vi "flashV6.vi"() -> ()   [LabVIEW 2017]
panel:
  in  "start":bool
  out "Current IP address":string
  in  "IP address list":string[](array[string])=["192.168.10.20", "192.168.10.22"]
  in  "回读":bool
  out "Current Progress":u32(slide)=3722240 scale=0.0..8559432.0
  out "error out":errorcluster={"status"=TRUE, "code"=4, "source"="Read from Binary File in flashV3.vi<APPEND>\nG:\\fpga_tdc\\FPGA\\TDC_2channel\\TOP.bin"}
  out "appended array":bool[](array[boolean])
  out "Process":u32=3722240
  in  "error in (no error)":errorcluster
  in  "Read (TRUE)":bool
  out "byte data":string
  out "Total size (in bytes)":i64=3722064
  in  "file path (use dialog)":path=path "G:/fpga_tdc/FPGA/SiTCP_410t/TDC_410t/TDC_410t.runs/impl_1/TOP.bin"
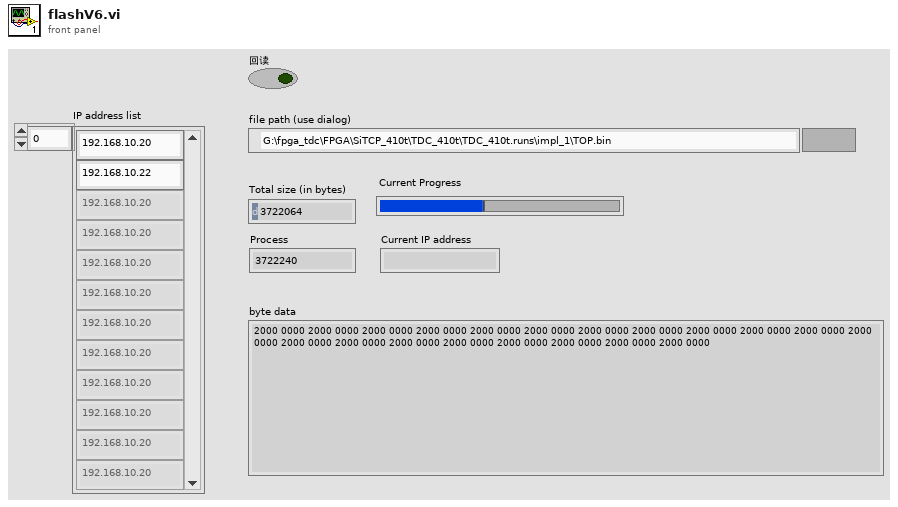
[diagram p1: front panel]
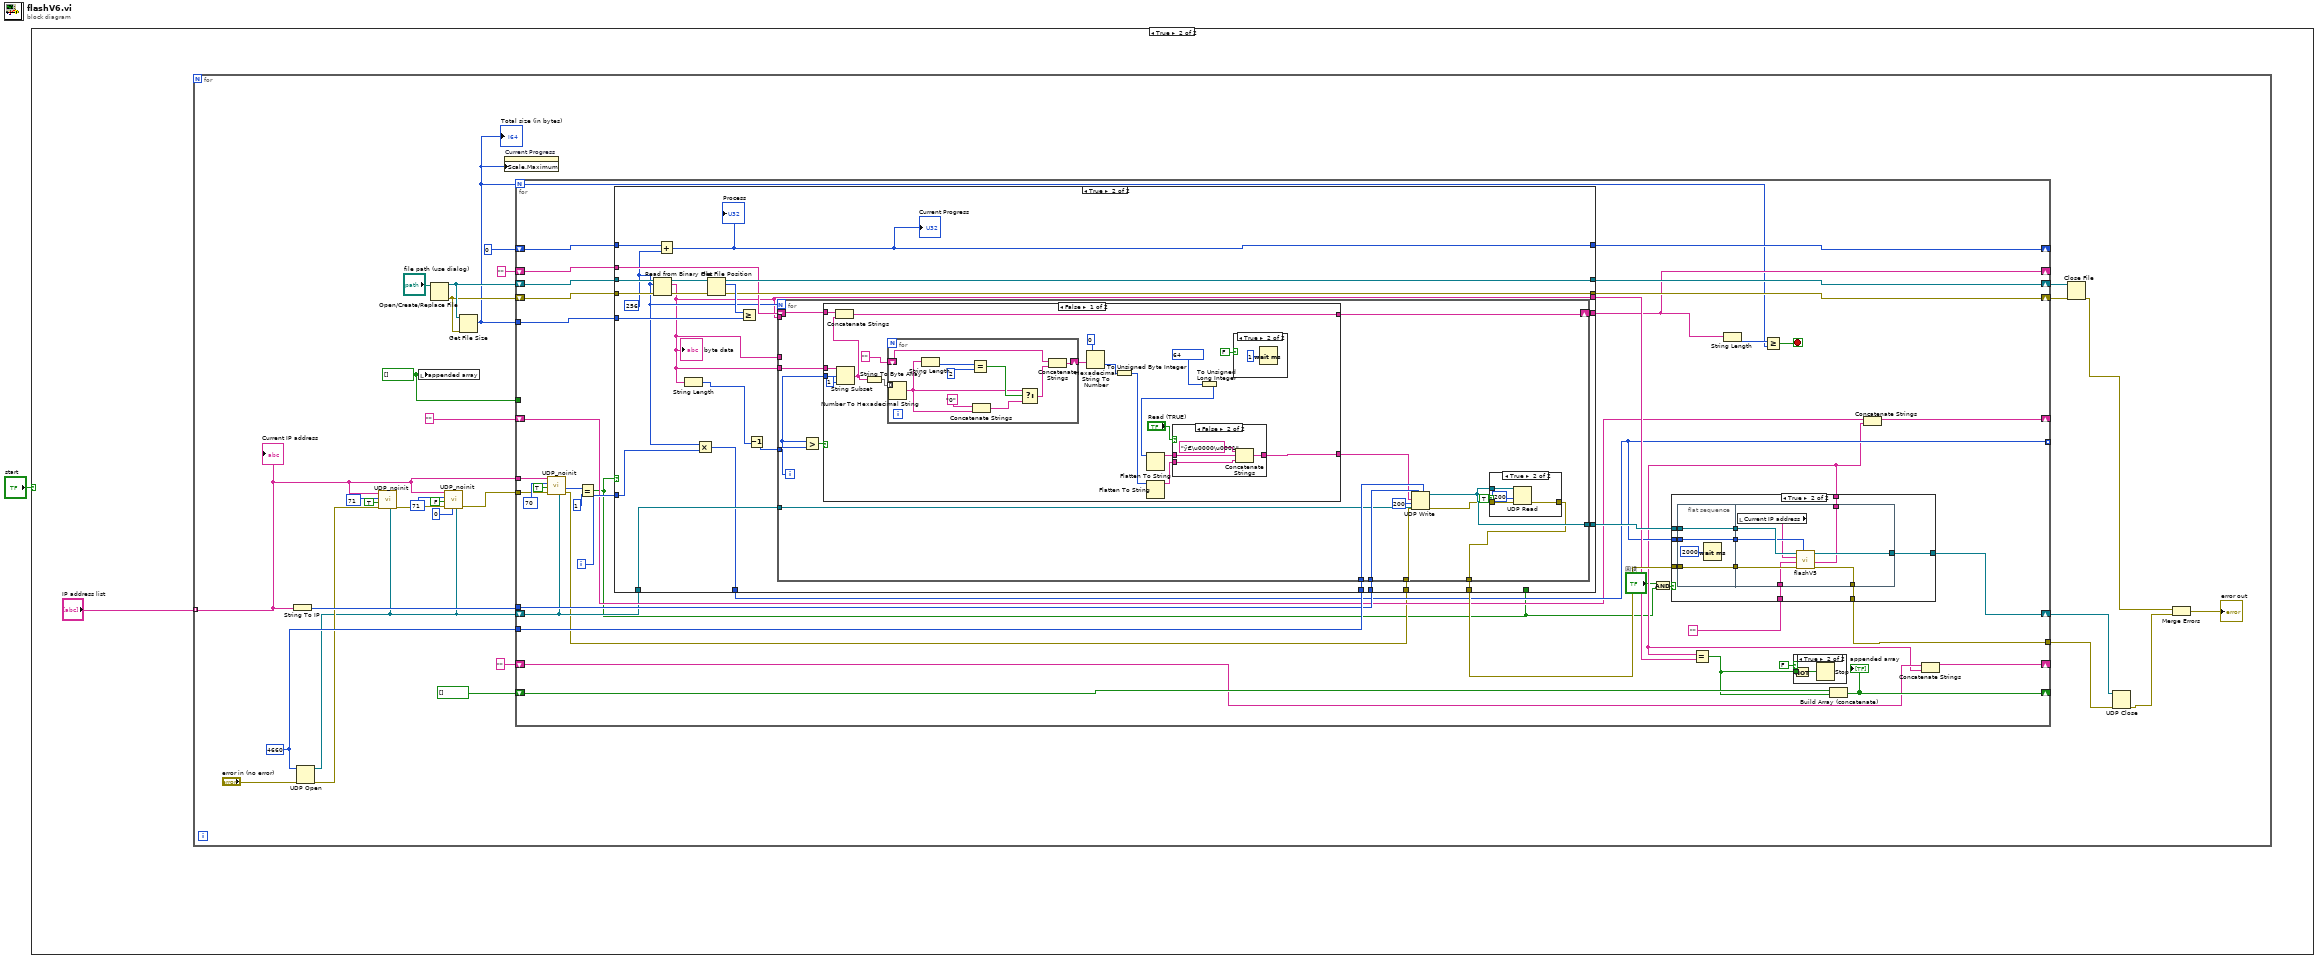
[diagram p0: block diagram]
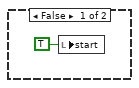
[diagram p2: hidden frame]
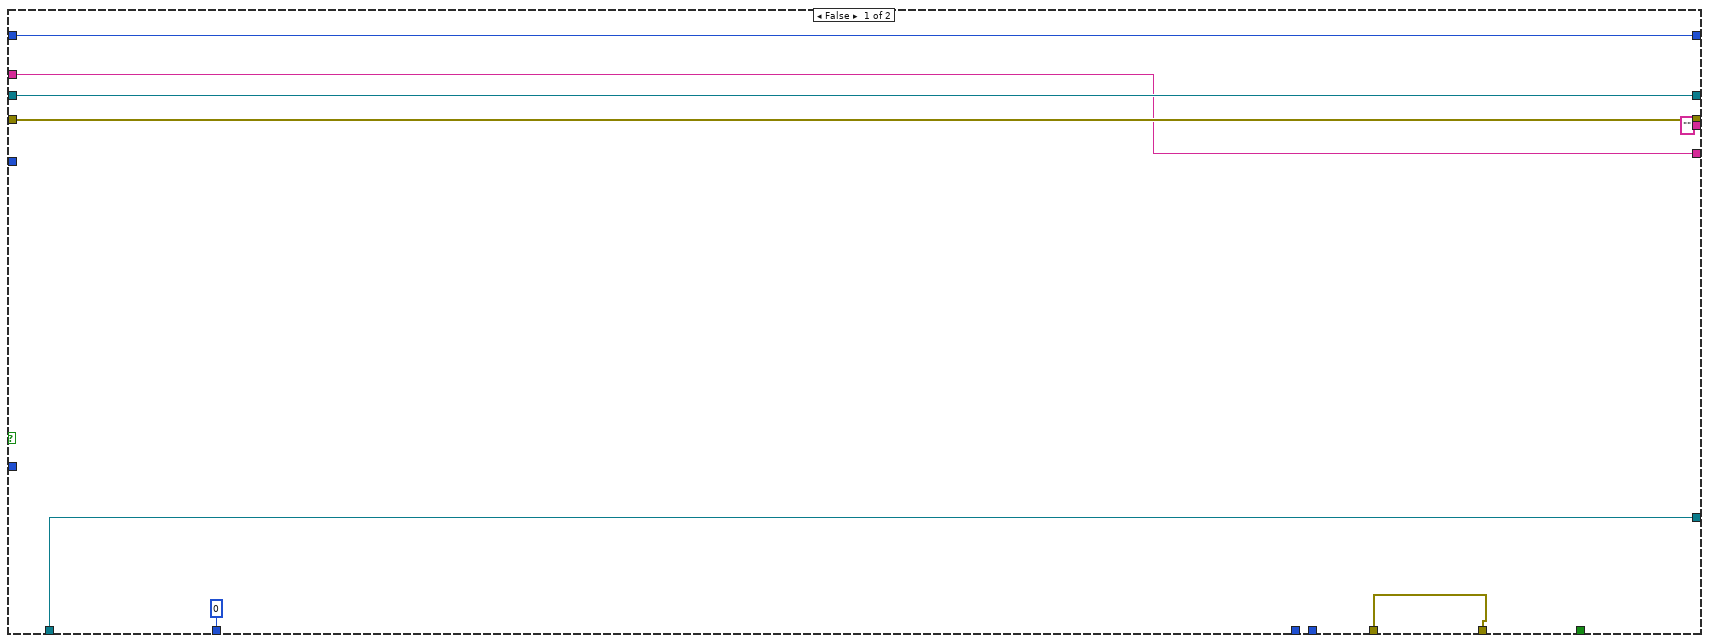
[diagram p3: hidden frame]
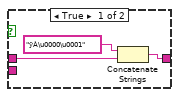
[diagram p5: hidden frame]
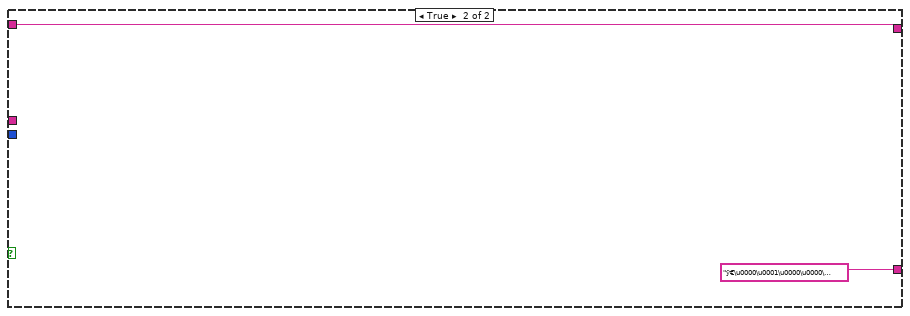
[diagram p7: hidden frame]
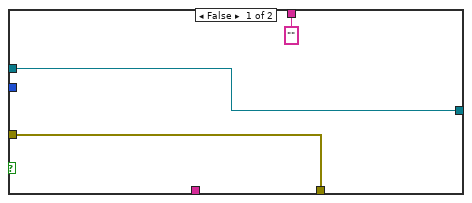
[diagram p8: hidden frame]
diagram:
  n1 = case shown="True" "start" {
    frame False {
      n2 = local write "start"(TRUE ("start")) -> ()
    }
    frame True {
      n3 = for {
        tunnel: "IP address list" -> [w13] mode=indexing
        w7 = bool[] [] ("appended array")
        w28 = u16 4660 ("UDP port")
        n4 = String To IP(1:w13) -> (0:w25:u32)
        n5 = UDP Open(8:"error in (no error)", 11:w28) -> (port=w10:refnum<k16>, 0:w15:errorcluster)  [unwired: 3 in, 1 out]
        n6 = call "UDP_noinit.vi"("connection ID"=w10, "error in (no error)"=w15, "Read (TRUE)"=TRUE, "Address"=u32 71, "IP address"=w13) -> ("error out"=w14:errorcluster)  [unwired: 3 in, 2 out]
        n7 = local write "appended array"(w7) -> ()
        n8 = Open/Create/Replace File(file path (use dialog)="file path (use dialog)") -> (refnum out=w32:refnum<file>, error out=w31:errorcluster)  [unwired: 5 in, 1 out]
        n9 = call "UDP_noinit.vi"("connection ID"=w10, "In"=u8 0, "error in (no error)"=w14, "Read (TRUE)"=FALSE, "Address"=u32 71, "IP address"=w13) -> ("error out"=w18:errorcluster)  [unwired: 2 in, 2 out]
        n10 = Get File Size(file=w32, error in=w31) -> (size (in bytes)=w8:i64)  [unwired: 2 out]
        "Total size (in bytes)" <- w8
        n11 = property on="Current Progress" class="Slide (strict)"("Scale.Maximum"=w8) -> ()  [unwired: 2 in, 2 out]
        n12 = for {
          N: w8 -> [w52]
          tunnel: w8 -> [w73]
          shift-right: [w72] -> w30
          shift-left: w31 -> [w74]
          shift-right: [w71] -> w29
          shift-left: w32 -> [w75]
          shift-right: [w54] -> _
          shift-left: "" -> [w70]
          tunnel: w28 -> [w67]
          tunnel: [w62] -> w26
          tunnel: w25 -> [w66]
          shift-right: [w64] -> w27
          shift-left: w10 -> [w41]
          shift-right: [w68] -> _
          shift-left: u32 0 ("length (rest)") -> [w69]
          shift-right: [w59] -> _
          shift-left: bool[] [] -> [w57]
          tunnel: [w55] -> _ mode=indexing
          shift-right: [w50] -> _
          shift-left: "" -> [w49]
          tunnel: w13 -> [w47]
          tunnel: w18 -> [w40]
          shift-right: [w38] -> _
          shift-left: "" -> [w37]
          tunnel: w7 -> [_]
          i -> [w60]
          stop <- w51 stop-if-true
          n13 = call "UDP_noinit.vi"("connection ID"=w41, "error in (no error)"=w40, "Read (TRUE)"=TRUE, "Address"=u32 70, "IP address"=w47) -> ("error out"=w39:errorcluster, "Out"=w44:u8)  [unwired: 3 in, 1 out]
          n14 = Equal?(x=w44, y=u8 1) -> (x = y?=w35:bool)
          n15 = case shown="True" w35 {
            tunnel: w75 -> [w80 w107]
            tunnel: w74 -> [w81 w106]
            tunnel: w73 -> [_ w102]
            tunnel: [w81 w101] -> w72
            tunnel: [w80 w100] -> w71
            tunnel: w70 -> [w78 w99]
            tunnel: w69 -> [w79 w98]
            tunnel: [w79 w84] -> w68
            tunnel: w67 -> [_ w97]
            tunnel: w66 -> [_ w96]
            tunnel: w39 -> [w82 w95]
            tunnel: w41 -> [w83 w94]
            tunnel: [w83 w91] -> w65
            tunnel: [w82 w90] -> w63
            tunnel: w60 -> [_ w89]
            tunnel: ["" w87] -> w58
            tunnel: [0 w86] -> w55
            tunnel: [w78 w85] -> w54
            tunnel: w35 -> [_ _]
            frame False {
            }
            frame True {
              w88 = 256 ("count (1)")
              n16 = Read from Binary File(8:w106, 10:w88, 11:w107) -> (0:w104:errorcluster, 2:w87:string, 3:w105:refnum<file>)  [unwired: 3 in, 1 out]
              "byte data" <- w87
              n17 = Add(x=w98, y=w88) -> (x+y=w84:u32)
              "Process" <- w84
              "Current Progress" <- w84
              n18 = String Length(string=w87) -> (length=w93:i32)
              n19 = Multiply(x=w88, y=w89) -> (x*y=w86:i32)
              n20 = Get File Position(4:w104, 7:w105) -> (0:w101:errorcluster, 2:w103:i64, 3:w100:refnum<file>)
              n21 = Greater Or Equal?(x=w103, y=w102) -> ()  [unwired: 1 out]
              n22 = Decrement(x=w93) -> (x-1=w92:i32)
              n23 = for {
                N: w88 -> [_]
                tunnel: w87 -> [_]
                tunnel: w87 -> [w123]
                tunnel: w87 -> [_]
                shift-right: [w121] -> w85
                shift-left: w99 -> [w122]
                tunnel: w97 -> [w120]
                tunnel: w96 -> [w119]
                tunnel: w95 -> [w118]
                tunnel: w94 -> [w112]
                tunnel: [w108] -> w90
                tunnel: [w111] -> w91
                tunnel: w92 -> [w115]
                i -> [w114]
                n24 = Greater?(x=w114, y=w115) -> (0:w116:bool)
                n25 = case shown="False" w116 {
                  tunnel: w123 -> [w139 _]
                  tunnel: w122 -> [w137 w166]
                  tunnel: [w136 w166] -> w121
                  tunnel: w114 -> [w130 _]
                  tunnel: [w129 "ÿ€\u0000\u0001\u0000\u0000\u0000@\u0000" ("字符串 2")] -> w113
                  frame False {
                    n26 = String Subset(string=w139, offset (0)=w130, length (rest)=1 ("length (rest)")) -> (substring=w135:string)
                    n27 = Concatenate Strings(w137, w135) -> (w136:string)
                    n28 = String To Byte Array(string=w135) -> (unsigned byte array=w146:u8[])
                    n29 = for {
                      shift-right: [w164] -> w145
                      shift-left: "" ("format string") -> [w161]
                      tunnel: w146 -> [w165] mode=indexing
                      n30 = Number To Hexadecimal String(2:w165) -> (0:w157:string)  [unwired: 1 in]
                      n31 = String Length(string=w157) -> (length=w163:i32)
                      n32 = Equal?(x=w163, y=2) -> (x = y?=w160:bool)
                      n33 = Concatenate Strings("0" ("format string"), w157) -> (w159:string)
                      n34 = Select(t=w157, s=w160, f=w159) -> (s? t:f=w156:string)
                      n35 = Concatenate Strings(w161, w156) -> (w164:string)
                    }
                    n36 = Hexadecimal String To Number(string=w145, default (0uL)=u64 0 ("default (0 U32)")) -> (number=w143:u64)  [unwired: 1 in, 1 out]
                    n37 = To Unsigned Byte Integer(number=w143) -> (unsigned 8bit integer=w141:u8)
                    n38 = Flatten To String(anything=w141) -> (data string=w132:string)  [unwired: 3 in, 2 out]
                    n39 = To Unsigned Long Integer(number=u32 64 ("Address")) -> (unsigned 32bit integer=w140:u32)
                    n40 = Flatten To String(anything=w140) -> (data string=w133:string)  [unwired: 3 in, 2 out]
                    n41 = case shown="False" "Read (TRUE)" {
                      tunnel: [w149 w153] -> w129
                      tunnel: w133 -> [w148 w152]
                      tunnel: w132 -> [_ w151]
                      frame True {
                        n42 = Concatenate Strings("ÿÀ\u0000\u0001" ("initial string"), w148) -> (w149:string)
                      }
                      frame False {
                        n43 = Concatenate Strings("ÿ€\u0000\u0001" ("initial string"), w152, w151) -> (w153:string)
                      }
                    }
                    n44 = case shown="True" FALSE {
                      frame False {
                      }
                      frame True {
                        n45 = Wait (ms)(milliseconds to wait=u32 1) -> ()  [unwired: 1 out]
                      }
                    }
                  }
                  frame True {
                  }
                }
                n46 = UDP Write(address=w119, port or service name=w120, connection ID=w112, data in=w113, 8:w118, 9:200 ("timeout ms (25000)")) -> (error out=w109:errorcluster, 3:w111:refnum<k16>)
                n47 = case shown="True" TRUE {
                  tunnel: w111 -> [_ w128]
                  tunnel: w109 -> [w124 w127]
                  tunnel: [w124 w126] -> w108
                  frame False {
                  }
                  frame True {
                    n48 = UDP Read(connection ID=w128, timeout ms (25000)=200, 8:w127) -> (error out=w126:errorcluster)  [unwired: 5 out]
                  }
                }
              }
            }
          }
          n49 = And(x="回读", y=w35) -> (x .and. y?=w42:bool)
          n50 = case shown="True" w42 {
            tunnel: w65 -> [w170 w177]
            tunnel: [w170 w176] -> w64
            tunnel: w63 -> [w169 w175]
            tunnel: [w169 w174] -> w62
            tunnel: "" ("empty") -> [_ w173]
            tunnel: w55 -> [_ w172]
            tunnel: ["" ("String") w171] -> w36
            frame False {
            }
            frame True {
              n51 = flat-sequence {
                tunnel: w172 -> [w182]
                tunnel: w175 -> [w183]
                tunnel: w177 -> [w184]
                tunnel: [w184] -> w180
                tunnel: [w183] -> w179
                tunnel: [w182] -> w178
                tunnel: [w189] -> w174
                tunnel: w173 -> [w188]
                tunnel: [w187] -> w171
                tunnel: w180 -> [w192]
                tunnel: w179 -> [w190]
                tunnel: w178 -> [w186]
                tunnel: [w191] -> w176
                frame #0 {
                  n52 = Wait (ms)(milliseconds to wait=u32 2000) -> ()  [unwired: 1 out]
                }
                frame #1 {
                  n53 = local read "Current IP address"() -> (w185:string)
                  n54 = call "flashV5.vi"("flash_base_address"=w186, "error in (no error)"=w190, "empty"=w188, "address"=w185, "connection ID"=w192) -> ("error out"=w189:errorcluster, "String"=w187:string, "connection ID 2"=w191:refnum<k16>)  [unwired: 3 in, 1 out]
                }
              }
            }
          }
          n55 = Equal?(x=w36, y=w58) -> (x = y?=w56:bool)
          n56 = String Length(string=w54) -> (length=w53:i32)
          n57 = Greater Or Equal?(x=w53, y=w52) -> (x >= y?=w51:bool)
          n58 = case shown="True" FALSE {
            tunnel: w56 -> [_ w193]
            frame False {
            }
            frame True {
              n59 = Not(x=w193) -> (.not. x?=w194:bool)
              n60 = Stop(stop? (T)=w194) -> ()
            }
          }
          n61 = Build Array (concatenate)(w57, w56) -> (w59:bool[])
          "appended array" <- w59
          n62 = Concatenate Strings(w49, w36) -> (w50:string)
          n63 = Concatenate Strings(w37, w36) -> (w38:string)
        }
        n64 = Close File(refnum=w29, error in=w30) -> (error out=w6:errorcluster)  [unwired: 1 out]
        n65 = UDP Close(connection ID=w27, 8:w26) -> (error out=w5:errorcluster)  [unwired: 1 out]
        n66 = Merge Errors(w6, w5) -> (→"error out":errorcluster)
        "Current IP address" <- w13
      }
    }
  }
